vi "诊断标定3 - 副本.vi"(8 "CAN端口":u16(ring), 9 "设备索引号":u16(ring), 10 "CAN卡类型":u32(ring)=21) -> ()   [LabVIEW 2013] (continued)
        }
        n2820 = Unbundle By Name(w898) -> ("status"=w897:bool)
        n2821 = Or(x=w897, y=w899) -> (x .or. y?=w900:bool)
      }
      n2822 = Release Queue(queue=w893, force destroy? (F)=TRUE ("强制销毁？(F)"), error in (no error)=w892) -> (error out=w890:errorcluster)  [unwired: 2 out]
      n2823 = call <vilib>:"Clear Errors.vi"("error in (no error)"=w890) -> ()  [unwired: 7 out]
    }
    frame Disabled {
    }
  }
  n2824 = while {
    tunnel: w36 -> [w3698]
    tunnel: w35 -> [w3697]
    tunnel: [w3696] -> w39
    tunnel: [w3695] -> w38
    tunnel: w31 -> [_]
    tunnel: w34 -> [w3687]
    stop <- w3694 stop-if-true
    n2825 = local read "停止"() -> (w3694:bool)
    n2826 = local read "设备索引号"() -> (w3691:u16)
    n2827 = local read "CAN卡类型"() -> (w3692:u32)
    n2828 = local read "CAN端口"() -> (w3690:u16)
    n2829 = call "receiver-8.6.vi"("错误输入（无错误）"=w3687, "CAN端口"=w3690, "设备索引号"=w3691, "CAN卡类型"=w3692) -> ("错误输出"=w3693:errorcluster, "输出簇"=w3689:T25, "接收成功"=w3688:bool)  [unwired: 3 out]
    n2830 = call <vilib>:"Clear Errors.vi"("error in (no error)"=w3693) -> ()  [unwired: 6 in, 1 out]
    n2831 = case shown="真" w3688 {
      tunnel: w3697 -> [w3699 w3705]
      tunnel: w3689 -> [_ w3704]
      tunnel: w3698 -> [w3700 w3703]
      tunnel: [w3700 w3702] -> w3696
      tunnel: [w3699 w3701] -> w3695
      frame False {
      }
      frame True {
        n2832 = Enqueue Element(queue=w3703, element=w3704, error in (no error)=w3705) -> (queue out=w3702:refnum<queue>, error out=w3701:errorcluster)  [unwired: 2 out]
      }
    }
  }
  n2833 = while {
    tunnel: w36 -> [w3713]
    tunnel: w35 -> [w3712]
    stop <- w3706 stop-if-true
    n2834 = local read "停止"() -> (w3706:bool)
    n2835 = local read "控制1"() -> (w3708:bool)
    n2836 = Dequeue Element(queue=w3713, timeout in ms (-1)=200 ("超时毫秒(-1)"), error in (no error)=w3712) -> (element=w3711:T3, error out=w3710:errorcluster)  [unwired: 2 out]
    n2837 = case shown="无错误" w3710 {
      tunnel: w3711 -> [w3718 _]
      tunnel: "写?" -> [w3715 _]
      tunnel: w3708 -> [w3714 _]
      frame No Error {
        n2838 = Unbundle(w3718) -> ("return type"=w3717:u32, "pReceive"=w3716:T26)
        n2839 = for {
          N: w3717 -> [_]
          tunnel: w3716 -> [w3722] mode=indexing
          tunnel: w3715 -> [w3720]
          tunnel: w3714 -> [w3719]
          n2840 = Unbundle By Name(w3722) -> ("ID"=w3723:u32)
          n2841 = call "ID解析.vi"("ID"=w3723) -> ("PDU(1)"=w3721:i32)  [unwired: 10 out]
          n2842 = case shown="18" w3721 {
            tunnel: w3722 -> [_ w3733]
            tunnel: w3720 -> [_ w3725]
            tunnel: w3719 -> [_ w3724]
            frame 0, Default {
            }
            frame 24 {
              n2843 = local read "主从选择"() -> (w3726:enum32{"主板", "从板"})
              n2844 = local read "设备索引号"() -> (w3729:u16)
              n2845 = local read "CAN卡类型"() -> (w3728:u32)
              n2846 = local read "CAN端口"() -> (w3730:u16)
              n2847 = disable-structure shown="禁用" {
                disable-tunnel: w3733 -> [w3736 _]
                frame Disabled {
                  n2848 = call "标定授权读取.vi"("VCI_Receive"=w3736) -> ()  [unwired: 1 out]
                }
                frame Enabled {
                }
              }
              n2849 = case shown="\"从板\"" w3726 {
                tunnel: [0 ("FUNC") w3735] -> w3727
                frame "主板", Default {
                }
                frame "从板" {
                  n2850 = local read "从板号"() -> (w3735:u8)
                }
              }
              n2851 = local read "面板选择"() -> (w3732:T7)
              n2852 = case shown="\"读写参数\", 默认" w3732 {
                tunnel: w3725 -> [w3741 _ _ _]
                tunnel: "命令" -> [w3742 w3841 w4096 w4236]
                tunnel: w3726 -> [w3751 _ w4104 w4244]
                tunnel: w3733 -> [_ _ _ _]
                tunnel: w3733 -> [w3747 w3842 w4098 w4238]
                tunnel: w3730 -> [w3746 w3843 w4099 w4239]
                tunnel: w3729 -> [w3745 w3844 w4100 w4240]
                tunnel: w3728 -> [w3744 w3845 w4101 w4241]
                tunnel: w3727 -> [w3743 _ w4097 w4237]
                tunnel: w3724 -> [w3737 _ _ _]
                frame "读写参数", Default {
                  n2853 = local read "命令序号"() -> (w3740:u8)
                  n2854 = call "多帧接收机制(EV05).vi"("can卡类型"=w3744, "设备索引号"=w3745, "CAN端口"=w3746, "VCI_Receive"=w3747, "命令"=w3742, "板号"=w3743, "写?"=w3741, "命令序号"=w3740) -> ("错误信号"=w3738:bool, "错误代码"=w3750:i32, "输出数组"=w3749:u8[], "读错误代码"=w3739:u8[], "结束信号"=w3748:bool)  [unwired: 7 out]
                  n2855 = case shown="假" w3741 {
                    tunnel: w3748 -> [w3761 w3824]
                    tunnel: w3750 -> [w3760 w3823]
                    tunnel: w3740 -> [w3759 _]
                    tunnel: w3749 -> [w3758 _]
                    tunnel: w3742 -> [w3757 _]
                    tunnel: w3751 -> [w3755 w3822]
                    tunnel: w3739 -> [w3754 _]
                    tunnel: w3738 -> [w3753 _]
                    tunnel: w3737 -> [w3752 _]
                    frame False {
                      # "读参数"
                      n2856 = And(x=w3752, y=w3761) -> (x .and. y?=w3756:bool)
                      n2857 = case shown="真" w3756 {
                        tunnel: w3760 -> [_ w3772]
                        tunnel: w3759 -> [_ w3771]
                        tunnel: w3758 -> [_ w3770]
                        tunnel: w3757 -> [_ w3769]
                        tunnel: w3755 -> [_ w3765]
                        tunnel: w3754 -> [_ w3763]
                        tunnel: w3753 -> [_ w3764]
                        frame False {
                        }
                        frame True {
                          n2858 = case shown="假" w3764 {
                            tunnel: w3772 -> [w3781 _]
                            tunnel: w3771 -> [w3780 _]
                            tunnel: w3770 -> [w3779 _]
                            tunnel: w3769 -> [w3777 _]
                            tunnel: w3765 -> [w3773 _]
                            tunnel: w3763 -> [_ w3807]
                            frame False {
                              n2859 = case shown="\"主板\", 默认" w3773 {
                                tunnel: [w3782 _] -> w3776
                                tunnel: [_ w3795] -> w3775
                                frame "主板", Default {
                                n2860 = stacked-sequence {
                                tunnel: [_ w3794] -> w3782
                                frame #0 {
                                n2861 = control-ref of="一级故障"() -> (w3788:refnum<vi>)
                                n2862 = control-ref of="一级故障 2"() -> (w3790:refnum<vi>)
                                n2863 = control-ref of="一级故障 3"() -> (w3791:refnum<vi>)
                                n2864 = control-ref of="加热控制参数"() -> (w3792:refnum<vi>)
                                n2865 = control-ref of="充电控制参数"() -> (w3793:refnum<vi>)
                                n2866 = control-ref of="电池信息"() -> (w3786:refnum<vi>)
                                n2867 = control-ref of="项目信息"() -> (w3789:refnum<vi>)
                                n2868 = control-ref of="项目信息2"() -> (w3787:refnum<vi>)
                                n2869 = control-ref of="高压参数"() -> (w3785:refnum<vi>)
                                n2870 = local read "主板数据"() -> (w3784:T4)
                                n2871 = Bundle(cluster=w3784, "项目信息"=w3789, "一级故障 4"=w3787, "一级故障"=w3788, "一级故障 2"=w3790, "一级故障 3"=w3791, "加热控制参数"=w3792, "充电控制参数"=w3793, "高压参数"=w3785, "电池信息"=w3786) -> (w3783:T4)
                                n2872 = local write "主板数据"(w3783) -> ()
                                }
                                frame #1 {
                                n2873 = control-ref of="主板数据"() -> (w3794:refnum<vi>)
                                }
                                }
                                }
                                frame "从板" {
                                n2874 = stacked-sequence {
                                tunnel: [_ w3806] -> w3795
                                frame #0 {
                                n2875 = control-ref of="从板号"() -> (w3800:refnum<vi>)
                                n2876 = control-ref of="项目信息 2"() -> (w3801:refnum<vi>)
                                n2877 = control-ref of="电池组信息"() -> (w3799:refnum<vi>)
                                n2878 = control-ref of="加热控制参数"() -> (w3802:refnum<vi>)
                                n2879 = control-ref of="一级故障(从板)"() -> (w3803:refnum<vi>)
                                n2880 = control-ref of="二级故障(从板)"() -> (w3804:refnum<vi>)
                                n2881 = control-ref of="三级故障(从板)"() -> (w3805:refnum<vi>)
                                n2882 = control-ref of="均衡参数"() -> (w3798:refnum<vi>)
                                n2883 = local read "从板信息"() -> (w3797:T2)
                                n2884 = Bundle(cluster=w3797, "从板号"=w3800, "项目信息 2"=w3801, "加热控制参数"=w3802, "一级故障(从板)"=w3803, "二级故障(从板)"=w3804, "三级故障(从板)"=w3805, "电池组信息(从板)"=w3799, "均衡参数"=w3798) -> (w3796:T2)
                                n2885 = local write "从板信息"(w3796) -> ()
                                }
                                frame #1 {
                                n2886 = control-ref of="从板信息"() -> (w3806:refnum<vi>)
                                }
                                }
                                }
                              }
                              n2887 = control-ref of="结果"() -> (w3778:refnum<vi>)
                              n2888 = control-ref of="从板个数"() -> (w3774:refnum<vi>)
                              n2889 = call "输出数据解析.vi"("主板引用"=w3776, "从板引用"=w3775, "板选择"=w3773, "错误代码"=w3781, "命令序号"=w3780, "输入数组"=w3779, "命令"=w3777, "进度引用"=w3778, "从板个数"=w3774) -> ()  [unwired: 2 in, 5 out]
                            }
                            frame True {
                              n2890 = Index Array(array=w3807, index #1=0 ("索引"), index #2=1 ("索引")) -> (element #1=w3810:u8, element #2=w3811:u8)
                              n2891 = Join Numbers(hi=w3810, lo=w3811) -> ((hi.lo)=w3809:u16)
                              n2892 = Number To Hexadecimal String(2:w3809) -> (0:w3808:string)  [unwired: 1 out]
                              n2893 = control-ref of="结果"() -> (w3816:refnum<vi>)
                              n2894 = Concatenate Strings("0x" ("字符串"), w3808) -> (w3817:string)
                              n2895 = Build Array(w3817) -> (w3818:string[])
                              n2896 = call "表格编辑.vi"("新元素/子数组"=w3818, "活动单元格:单元格背景色"=u32 16740749, "MCListbox引用句柄"=w3816) -> ()  [unwired: 9 out]
                            }
                          }
                          n2897 = global write "EV05全局变量1.vi" "流控帧 2"(FALSE ("流控帧 2")) -> ()
                          n2898 = global write "EV05全局变量1.vi" "输出数组"(i32[] []) -> ()
                          n2899 = local write "控制1"(FALSE ("控制1")) -> ()
                          n2900 = local write "消除"(FALSE ("消除")) -> ()
                        }
                      }
                    }
                    frame True {
                      # "写参数判定"
                      n2901 = And(x="控制1", y=w3824) -> (x .and. y?=w3821:bool)
                      n2902 = case shown="真" w3821 {
                        tunnel: w3823 -> [_ w3831]
                        tunnel: w3822 -> [_ w3828]
                        frame False {
                        }
                        frame True {
                          n2903 = call <vilib>:"Unset Busy.vi"() -> ()  [unwired: 2 in, 10 out]
                          n2904 = case shown="\"从板\"" w3828 {
                            tunnel: [w3832 w3833] -> w3830
                            frame "主板", Default {
                              n2905 = local read "主板选项"() -> (w3832:string)
                            }
                            frame "从板" {
                              n2906 = local read "从板选项"() -> (w3833:string)
                            }
                          }
                          n2907 = control-ref of="结果"() -> (w3829:refnum<vi>)
                          n2908 = call "输入数据判定.vi"("主从选择"=w3828, "主板选项"=w3830, "进度引用"=w3829, "错误代码"=w3831) -> ()  [unwired: 2 in, 6 out]
                          n2909 = global write "EV05全局变量1.vi" "流控帧 2"(FALSE ("流控帧 2")) -> ()
                          n2910 = local write "控制1"(FALSE ("控制1")) -> ()
                          n2911 = local write "消除"(FALSE ("消除")) -> ()
                        }
                      }
                      n2912 = global write "EV05全局变量1.vi" "输出数组"(i32[] []) -> ()
                    }
                  }
                }
                frame "版本读取" {
                  n2913 = local read "命令序号"() -> (w3834:u8)
                  n2914 = local read "从板板号"() -> (w3837:u8)
                  n2915 = local read "控制1"() -> (w3838:bool)
                  n2916 = call "多帧接收机制(EV05).vi"("can卡类型"=w3845, "设备索引号"=w3844, "CAN端口"=w3843, "VCI_Receive"=w3842, "命令"=w3841, "板号"=w3837, "命令序号"=w3834) -> ("错误信号"=w3835:bool, "输出数组"=w3846:u8[], "读错误代码"=w3836:u8[], "结束信号"=w3840:bool)  [unwired: 1 in, 8 out]
                  n2917 = And(x=w3838, y=w3840) -> (x .and. y?=w3839:bool)
                  n2918 = case shown="真" w3839 {
                    tunnel: w3846 -> [_ w3854]
                    tunnel: w3834 -> [_ w3853]
                    tunnel: w3841 -> [_ w3852]
                    tunnel: w3836 -> [_ w3848]
                    tunnel: w3835 -> [_ w3847]
                    frame False {
                    }
                    frame True {
                      n2919 = case shown="假" w3847 {
                        tunnel: w3854 -> [w3858 _]
                        tunnel: w3853 -> [w3857 _]
                        tunnel: w3852 -> [w3856 _]
                        tunnel: w3848 -> [w3855 w4082]
                        frame False {
                          n2920 = case shown="89" w3856 {
                            tunnel: w3857 -> [_ w3861]
                            tunnel: w3858 -> [_ w3860]
                            tunnel: w3855 -> [_ _]
                            frame 0, Default {
                            }
                            frame 137 {
                              n2921 = case shown="1" w3861 {
                                tunnel: w3860 -> [_ w3889 w3933 w3953 w4080]
                                frame 0, Default {
                                }
                                frame 1 {
                                w3871 = "." ("字符串")
                                n2922 = Array Subset(array=w3889, index=0 ("索引"), length=14 ("长度")) -> (w3902:u8[])
                                n2923 = Index Array(array=w3889, index=14 ("索引")) -> (element=w3892:u8)
                                n2924 = Index Array(array=w3889, index #1=15 ("索引"), index #2=16 ("索引")) -> (element #1=w3898:u8, element #2=w3899:u8)
                                n2925 = Index Array(array=w3889, index #1=17 ("索引"), index #2=18 ("索引")) -> (element #1=w3893:u8, element #2=w3894:u8)
                                n2926 = call "数组去零.vi"("输入"=w3902) -> ("输出"=w3877:dbl[])
                                n2927 = Join Numbers(hi=w3893, lo=w3894) -> ((hi.lo)=w3890:u16)
                                n2928 = Join Numbers(hi=w3898, lo=w3899) -> ((hi.lo)=w3891:u16)
                                n2929 = Number To Decimal String(number=w3892) -> (decimal integer string=w3884:string)  [unwired: 1 out]
                                n2930 = Byte Array To String(unsigned byte array=w3877) -> (string=w3876:string)
                                n2931 = Number To Decimal String(number=w3890) -> (decimal integer string=w3872:string)  [unwired: 1 out]
                                n2932 = Number To Decimal String(number=w3891) -> (decimal integer string=w3883:string)  [unwired: 1 out]
                                n2933 = Array Subset(array=w3889, index=21 ("索引"), length=7 ("长度")) -> (w3886:u8[])
                                n2934 = Concatenate Strings("V" ("字符串"), w3884, w3871, w3883, w3871, w3872) -> (w3881:string)
                                n2935 = call "数组去零.vi"("输入"=w3886) -> ("输出"=w3869:dbl[])
                                n2936 = Byte Array To String(unsigned byte array=w3869) -> (string=w3867:string)
                                n2937 = call <vilib>:"Space Constant.vi"() -> ("String"=w3868:string)
                                n2938 = Equal?(x=w3867, y=w3868) -> (x = y?=w3873:bool)
                                n2939 = Concatenate Strings("-" ("字符串"), w3867) -> (w3874:string)
                                n2940 = Select(t=w3868, s=w3873, f=w3874) -> (s? t:f=w3870:string)
                                n2941 = Concatenate Strings(w3876, "-" ("字符串"), w3881, w3870) -> (w3863:string)
                                n2942 = local read "项目软件版本"() -> (w3865:string[])
                                n2943 = local read "从板板号"() -> (w3862:u8)
                                n2944 = local write "项目软件版本号"(w3863) -> ()
                                n2945 = Replace Array Subset(array=w3865, new element=w3863, index=w3862) -> (w3864:string[])
                                n2946 = control-ref of="结果"() -> (w3880:refnum<vi>)
                                n2947 = local write "项目软件版本"(w3864) -> ()
                                n2948 = Build Array("项目软件版本     读取完成" ("读取结果")) -> (w3878:string[])
                                n2949 = call "表格编辑(版本读取).vi"("新元素/子数组"=w3878, "活动单元格:单元格背景色"=u32 6618880, "MCListbox引用句柄"=w3880) -> ()  [unwired: 9 out]
                                }
                                frame 2 {
                                w3916 = ""
                                w3913 = "." ("字符串")
                                n2950 = Array Subset(array=w3933, index=0 ("索引"), length=14 ("长度")) -> (w3921:u8[])
                                n2951 = Index Array(array=w3933, index=14 ("索引")) -> (element=w3936:u8)
                                n2952 = Index Array(array=w3933, index #1=15 ("索引"), index #2=16 ("索引")) -> (element #1=w3942:u8, element #2=w3943:u8)
                                n2953 = Index Array(array=w3933, index #1=17 ("索引"), index #2=18 ("索引")) -> (element #1=w3937:u8, element #2=w3938:u8)
                                n2954 = Join Numbers(hi=w3937, lo=w3938) -> ((hi.lo)=w3934:u16)
                                n2955 = Join Numbers(hi=w3942, lo=w3943) -> ((hi.lo)=w3935:u16)
                                n2956 = Number To Decimal String(number=w3934) -> (decimal integer string=w3914:string)  [unwired: 1 out]
                                n2957 = call "数组去零.vi"("输入"=w3921) -> ("输出"=w3920:dbl[])
                                n2958 = Number To Decimal String(number=w3936) -> (decimal integer string=w3928:string)  [unwired: 1 out]
                                n2959 = Number To Decimal String(number=w3935) -> (decimal integer string=w3927:string)  [unwired: 1 out]
                                n2960 = Array Subset(array=w3933, index=21 ("索引"), length=7 ("长度")) -> (w3930:u8[])
                                n2961 = Byte Array To String(unsigned byte array=w3920) -> (string=w3915:string)
                                n2962 = call "数组去零.vi"("输入"=w3930) -> ("输出"=w3912:dbl[])
                                n2963 = Concatenate Strings("V" ("字符串"), w3928, w3913, w3927, w3913, w3914) -> (w3925:string)
                                n2964 = Byte Array To String(unsigned byte array=w3912) -> (string=w3910:string)
                                n2965 = Equal?(x=w3916, y=w3910) -> (x = y?=w3917:bool)
                                n2966 = Concatenate Strings("-" ("字符串"), w3910) -> (w3918:string)
                                n2967 = Select(t=w3916, s=w3917, f=w3918) -> (s? t:f=w3911:string)
                                n2968 = Concatenate Strings(w3915, "-" ("字符串"), w3925, w3911) -> (w3906:string)
                                n2969 = local read "平台软件版本"() -> (w3908:string[])
                                n2970 = local read "从板板号"() -> (w3905:u8)
                                n2971 = local write "平台软件版本号"(w3906) -> ()
                                n2972 = Replace Array Subset(array=w3908, new element=w3906, index=w3905) -> (w3907:string[])
                                n2973 = control-ref of="结果"() -> (w3923:refnum<vi>)
                                n2974 = local write "平台软件版本"(w3907) -> ()
                                n2975 = Build Array("平台软件版本     读取完成" ("读取结果")) -> (w3922:string[])
                                n2976 = call "表格编辑(版本读取).vi"("新元素/子数组"=w3922, "活动单元格:单元格背景色"=u32 6618880, "MCListbox引用句柄"=w3923) -> ()  [unwired: 1 in, 8 out]
                                }
                                frame 3 {
                                n2977 = Index Array(array=w3953, index #1=0 ("索引"), index #2=1 ("索引")) -> (element #1=w3949:u8, element #2=w3950:u8)
                                n2978 = Join Numbers(hi=w3949, lo=w3950) -> ((hi.lo)=w3948:u16)
                                n2979 = case shown="99, 默认" w3948 {
                                tunnel: w3953 -> [w3956 _ w3990]
                                tunnel: w3948 -> [_ _ w3968]
                                frame 0 {
                                n2980 = Index Array(array=w3956, index #1=2 ("索引"), index #2=3 ("索引")) -> (element #1=w3960:u8, element #2=w3959:u8)
                                n2981 = Join Numbers(hi=w3960, lo=w3959) -> ((hi.lo)=w3955:u16)
                                n2982 = for {
                                N: w3955 -> [_]
                                tunnel: w3956 -> [w3965]
                                tunnel: [w3961] -> w3954 mode=indexing
                                i -> [w3964]
                                n2983 = Add(x=w3964, y=4) -> (x+y=w3962:i32)
                                n2984 = Index Array(array=w3965, index=w3962) -> (element=w3961:u8)
                                }
                                "MODEL号" <- w3954
                                }
                                frame 99, Default {
                                }
                                frame 1..40 {
                                w3973 = ""
                                w3994 = "." ("字符串")
                                n2985 = Array Subset(array=w3990, index=2 ("索引"), length=14 ("长度")) -> (w3979:u8[])
                                n2986 = Index Array(array=w3990, index=16 ("索引")) -> (element=w4002:u8)
                                n2987 = Index Array(array=w3990, index #1=17 ("索引"), index #2=18 ("索引")) -> (element #1=w4008:u8, element #2=w4009:u8)
                                n2988 = Index Array(array=w3990, index #1=19 ("索引"), index #2=20 ("索引")) -> (element #1=w4003:u8, element #2=w4004:u8)
                                n2989 = Join Numbers(hi=w4003, lo=w4004) -> ((hi.lo)=w4000:u16)
                                n2990 = Join Numbers(hi=w4008, lo=w4009) -> ((hi.lo)=w4001:u16)
                                n2991 = Number To Decimal String(number=w3968) -> (decimal integer string=w3988:string)  [unwired: 1 out]
                                n2992 = Number To Decimal String(number=w4002) -> (decimal integer string=w3996:string)  [unwired: 1 out]
                                n2993 = call "数组去零.vi"("输入"=w3979) -> ("输出"=w3978:dbl[])
                                n2994 = Number To Decimal String(number=w4001) -> (decimal integer string=w3995:string)  [unwired: 1 out]
                                n2995 = Number To Decimal String(number=w4000) -> (decimal integer string=w3993:string)  [unwired: 1 out]
                                n2996 = Byte Array To String(unsigned byte array=w3978) -> (string=w3980:string)
                                n2997 = Concatenate Strings("第" ("读取结果"), w3988, "模块" ("字符串"), "     读取完成" ("读取结果")) -> (w3981:string)
                                n2998 = Concatenate Strings("V" ("字符串"), w3996, w3994, w3995, w3994, w3993) -> (w3991:string)
                                n2999 = control-ref of="结果"() -> (w3984:refnum<vi>)
                                n3000 = Array Subset(array=w3990, index=23 ("索引"), length=7 ("长度")) -> (w3977:u8[])
                                n3001 = call "数组去零.vi"("输入"=w3977) -> ("输出"=w3972:dbl[])
                                n3002 = Byte Array To String(unsigned byte array=w3972) -> (string=w3969:string)
                                n3003 = Build Array(w3981) -> (w3983:string[])
                                n3004 = control-ref of="模块软件版本 2"() -> (w3985:refnum<vi>)
                                n3005 = local read "模块软件版本"() -> (w3986:T1)
                                n3006 = Equal?(x=w3973, y=w3969) -> (x = y?=w3974:bool)
                                n3007 = call "表格编辑(版本读取).vi"("新元素/子数组"=w3983, "活动单元格:单元格背景色"=u32 6618880, "MCListbox引用句柄"=w3984) -> ()  [unwired: 1 in, 8 out]
                                n3008 = Concatenate Strings("-" ("字符串"), w3969) -> (w3975:string)
                                n3009 = Select(t=w3973, s=w3974, f=w3975) -> (s? t:f=w3971:string)
                                n3010 = Concatenate Strings(w3980, "-" ("字符串"), w3991, w3971) -> (w3970:string)
                                n3011 = case shown="30" w3968 {
                                tunnel: [_ "VERSIONM" "BCUMCAL" "BMUMCAL" "BMURMCAL" "BCUCMCAL" "BCUDMCAL" "SCH" "BSW" "CDD" "DATALAYER" "DATAANALYSIS" "SOC" "SOH" "SOF" "INTRES" "INTCAN" "CARCAN" "CHGCANL" "THM" "CHGM" "HVM" "LVM" "BALM" "SAFEM" "RUNMODEM" "RELAY" "DO" "GBCHGDET" "SUPPLYPOWGDET" "SUMVDET" "CURDET" "TEMPERDET" "CELLVDET" "ISODET" "AI" "DI" "SYSCONF" "ECUCONF"] -> w3967
                                frame 0, Default {
                                }
                                frame 1 {
                                }
                                frame 2 {
                                }
                                frame 3 {
                                }
                                frame 4 {
                                }
                                frame 5 {
                                }
                                frame 6 {
                                }
                                frame 7 {
                                }
                                frame 8 {
                                }
                                frame 9 {
                                }
                                frame 10 {
                                }
                                frame 11 {
                                }
                                frame 12 {
                                }
                                frame 13 {
                                }
                                frame 14 {
                                }
                                frame 15 {
                                }
                                frame 16 {
                                }
                                frame 17 {
                                }
                                frame 18 {
                                }
                                frame 19 {
                                }
                                frame 20 {
                                }
                                frame 21 {
                                }
                                frame 22 {
                                }
                                frame 23 {
                                }
                                frame 24 {
                                }
                                frame 25 {
                                }
                                frame 26 {
                                }
                                frame 27 {
                                }
                                frame 28 {
                                }
                                frame 29 {
                                }
                                frame 30 {
                                }
                                frame 31 {
                                }
                                frame 32 {
                                }
                                frame 33 {
                                }
                                frame 34 {
                                }
                                frame 35 {
                                }
                                frame 36 {
                                }
                                frame 37 {
                                }
                                frame 38 {
                                }
                                }
                                n3012 = case shown="\"全部读取\"" w3986 {
                                tunnel: w3970 -> [w4053 w4061]
                                tunnel: w3968 -> [w4057 w4066]
                                tunnel: w3985 -> [w4059 w4067]
                                tunnel: w3967 -> [w4058 w4065]
                                frame "全部读取" {
                                n3013 = Number To Decimal String(number=w4057) -> (decimal integer string=w4056:string)  [unwired: 1 out]
                                n3014 = Concatenate Strings(w4056, "-" ("元素"), w4058) -> (w4054:string)
                                n3015 = Build Array(w4054, w4053) -> (w4052:string[])
                                n3016 = call "表格编辑(模块版本).vi"("新元素/子数组"=w4052, "MCListbox引用句柄"=w4059) -> ()  [unwired: 1 in, 9 out]
                                }
                                frame "BCUMCAL", Default {
                                n3017 = Number To Decimal String(number=w4066) -> (decimal integer string=w4064:string)  [unwired: 1 out]
                                n3018 = Concatenate Strings(w4064, "-" ("元素"), w4065) -> (w4062:string)
                                n3019 = Build Array(w4062, w4061) -> (w4060:string[])
                                n3020 = call "表格编辑(模块版本).vi"("新元素/子数组"=w4060, "MCListbox引用句柄"=w4067) -> ()  [unwired: 1 in, 9 out]
                                }
                                }
                                }
                                }
                                }
                                frame 4 {
                                n3021 = Array Subset(array=w4080, length=12 ("长度")) -> (w4078:u8[])  [unwired: 1 in]
                                n3022 = Byte Array To String(unsigned byte array=w4078) -> (string=w4077:string)
                                n3023 = call <vilib>:"Trim Whitespace.vi"("string"=w4077) -> ("trimmed string"=w4069:string)  [unwired: 1 in]
                                n3024 = local read "从板板号"() -> (w4068:u8)
                                n3025 = local write "硬件版本号"(w4069) -> ()
                                n3026 = local read "硬件版本"() -> (w4070:string[])
                                n3027 = Replace Array Subset(array=w4070, new element=w4069, index=w4068) -> (w4071:string[])
                                n3028 = local write "硬件版本"(w4071) -> ()
                                n3029 = global write "EV05全局变量1.vi" "写入超时"(TRUE ("写入超时")) -> ()
                                n3030 = control-ref of="结果"() -> (w4075:refnum<vi>)
                                n3031 = Build Array("硬件版本     读取完成" ("读取结果")) -> (w4074:string[])
                                n3032 = call "表格编辑(版本读取).vi"("新元素/子数组"=w4074, "活动单元格:单元格背景色"=u32 6618880, "MCListbox引用句柄"=w4075) -> ()  [unwired: 9 out]
                                }
                              }
                              n3033 = global write "EV05全局变量1.vi" "写入超时"(TRUE ("写入超时")) -> ()
                            }
                          }
                        }
                        frame True {
                          n3034 = Index Array(array=w4082, index #1=0 ("索引"), index #2=1 ("索引")) -> (element #1=w4087:u8, element #2=w4088:u8)
                          n3035 = Join Numbers(hi=w4087, lo=w4088) -> ((hi.lo)=w4086:u16)
                          n3036 = Number To Hexadecimal String(2:w4086) -> (0:w4085:string)  [unwired: 1 out]
                          n3037 = control-ref of="结果"() -> (w4084:refnum<vi>)
                          n3038 = Concatenate Strings("0x" ("字符串"), w4085) -> (w4092:string)
                          n3039 = Build Array(w4092) -> (w4083:string[])
                          n3040 = call "表格编辑(版本读取).vi"("新元素/子数组"=w4083, "活动单元格:单元格背景色"=u32 16740749, "MCListbox引用句柄"=w4084) -> ()  [unwired: 9 out]
                        }
                      }
                      n3041 = global write "EV05全局变量1.vi" "流控帧 2"(FALSE ("流控帧 2")) -> ()
                      n3042 = local write "控制1"(FALSE ("控制1")) -> ()
                      n3043 = local write "消除"(FALSE ("消除")) -> ()
                      n3044 = call <vilib>:"Unset Busy.vi"() -> ()  [unwired: 2 in, 10 out]
                    }
                  }
                }
                frame "其它诊断" {
                  n3045 = local read "命令序号"() -> (w4094:u8)
                  n3046 = call "多帧接收机制(EV05).vi"("can卡类型"=w4101, "设备索引号"=w4100, "CAN端口"=w4099, "VCI_Receive"=w4098, "命令"=w4096, "板号"=w4097, "命令序号"=w4094) -> ("错误代码"=w4103:i32, "输出数组"=w4095:u8[], "读错误代码"=w4093:u8[], "结束信号"=w4102:bool)  [unwired: 1 in, 8 out]
                  n3047 = case shown="真" w4102 {
                    tunnel: w4104 -> [_ w4105]
                    tunnel: w4103 -> [_ _]
                    tunnel: w4095 -> [_ w4106]
                    tunnel: w4094 -> [_ w4109]
                    tunnel: w4093 -> [_ w4107]
                    frame False {
                    }
                    frame True {
                      n3048 = Insert Into Array(array=w4107, new element=w4106) -> (w4108:u8[])  [unwired: 1 in]
                      n3049 = case shown="1" w4109 {
                        tunnel: w4108 -> [_ w4118 w4204]
                        tunnel: w4105 -> [_ _ w4199]
                        frame 0, Default {
                        }
                        frame 1 {
                          n3050 = Index Array(array=w4118) -> (element #1=w4117:u8, element #2=w4116:u8, element #3=w4115:u8)  [unwired: 3 in]
                          n3051 = Join Numbers(hi=w4116, lo=w4115) -> ((hi.lo)=w4114:u16)
                          n3052 = case shown="4" w4117 {
                            tunnel: w4118 -> [_ _ _ _ _ _ _ _ _ _]
                            tunnel: w4114 -> [_ w4121 w4129 w4139 w4149 w4159 w4169 w4179 w4189 _]
                            frame 0, Default {
                              n3053 = local write "继电器超时处理"(FALSE ("继电器超时处理")) -> ()
                            }
                            frame 1 {
                              n3054 = Equal To 0?(x=w4121) -> (x = 0?=w4120:bool)
                              n3055 = local write "正级继电器 12"(w4120) -> ()
                              n3056 = case shown="假" w4120 {
                                tunnel: w4121 -> [w4124 _]
                                frame False {
                                n3057 = local read "正级继电器"() -> (w4126:bool)
                                n3058 = Number To Hexadecimal String(2:w4124) -> (0:w4123:string)  [unwired: 1 out]
                                n3059 = local write "继电器超时处理"(TRUE ("继电器超时处理")) -> ()
                                n3060 = Not(x=w4126) -> (.not. x?=w4125:bool)
                                n3061 = Concatenate Strings("继电器操作失败,0x" ("消息"), w4123) -> ()  [unwired: 1 out]
                                n3062 = local write "正级继电器"(w4125) -> ()
                                }
                                frame True {
                                (unwired) "继电器操作成功!\n继电器操作成功!\n继电器操作成功!"
                                }
                              }
                            }
                            frame 2 {
                              n3063 = Equal To 0?(x=w4129) -> (x = 0?=w4128:bool)
                              n3064 = case shown="假" w4128 {
                                tunnel: w4129 -> [w4135 _]
                                tunnel: [w4133 "继电器操作成功!\n继电器操作成功!\n继电器操作成功!"] -> _
                                frame False {
                                n3065 = local read "负级继电器"() -> (w4131:bool)
                                n3066 = Number To Hexadecimal String(2:w4135) -> (0:w4134:string)  [unwired: 1 out]
                                n3067 = local write "继电器超时处理"(TRUE ("继电器超时处理")) -> ()
                                n3068 = Not(x=w4131) -> (.not. x?=w4132:bool)
                                n3069 = Concatenate Strings("继电器操作失败,0x" ("消息"), w4134) -> (w4133:string)
                                n3070 = local write "负级继电器"(w4132) -> ()
                                }
                                frame True {
                                }
                              }
                              n3071 = local write "正级继电器 2"(w4128) -> ()
                            }
                            frame 3 {
                              n3072 = Equal To 0?(x=w4139) -> (x = 0?=w4138:bool)
                              n3073 = case shown="假" w4138 {
                                tunnel: w4139 -> [w4145 _]
                                tunnel: [w4143 "继电器操作成功!\n继电器操作成功!\n继电器操作成功!"] -> _
                                frame False {
                                n3074 = local read "预充电继电器"() -> (w4141:bool)
                                n3075 = Number To Hexadecimal String(2:w4145) -> (0:w4144:string)  [unwired: 1 out]
                                n3076 = local write "继电器超时处理"(TRUE ("继电器超时处理")) -> ()
                                n3077 = Not(x=w4141) -> (.not. x?=w4142:bool)
                                n3078 = Concatenate Strings("继电器操作失败,0x" ("消息"), w4144) -> (w4143:string)
                                n3079 = local write "预充电继电器"(w4142) -> ()
                                }
                                frame True {
                                }
                              }
                              n3080 = local write "正级继电器 3"(w4138) -> ()
                            }
                            frame 4 {
                              n3081 = Equal To 0?(x=w4149) -> (x = 0?=w4148:bool)
                              n3082 = case shown="假" w4148 {
                                tunnel: w4149 -> [w4155 _]
                                tunnel: [w4153 "继电器操作成功!\n继电器操作成功!\n继电器操作成功!"] -> _
                                frame False {
                                n3083 = local read "加热继电器"() -> (w4152:bool)
                                n3084 = Number To Hexadecimal String(2:w4155) -> (0:w4154:string)  [unwired: 1 out]
                                n3085 = local write "继电器超时处理"(TRUE ("继电器超时处理")) -> ()
                                n3086 = Not(x=w4152) -> (.not. x?=w4151:bool)
                                n3087 = Concatenate Strings("继电器操作失败,0x" ("消息"), w4154) -> (w4153:string)
                                n3088 = local write "加热继电器"(w4151) -> ()
                                }
                                frame True {
                                }
                              }
                              n3089 = local write "正级继电器 5"(w4148) -> ()
                            }
                            frame 5 {
                              n3090 = Equal To 0?(x=w4159) -> (x = 0?=w4158:bool)
                              n3091 = case shown="假" w4158 {
                                tunnel: w4159 -> [w4165 _]
                                tunnel: [w4163 "继电器操作成功!\n继电器操作成功!\n继电器操作成功!"] -> _
                                frame False {
                                n3092 = local read "充电继电器"() -> (w4161:bool)
                                n3093 = Number To Hexadecimal String(2:w4165) -> (0:w4164:string)  [unwired: 1 out]
                                n3094 = local write "继电器超时处理"(TRUE ("继电器超时处理")) -> ()
                                n3095 = Not(x=w4161) -> (.not. x?=w4162:bool)
                                n3096 = Concatenate Strings("继电器操作失败,0x" ("消息"), w4164) -> (w4163:string)
                                n3097 = local write "充电继电器"(w4162) -> ()
                                }
                                frame True {
                                }
                              }
                              n3098 = local write "正级继电器 4"(w4158) -> ()
                            }
                            frame 6 {
                              n3099 = Equal To 0?(x=w4169) -> (x = 0?=w4168:bool)
                              n3100 = local write "正级继电器 6"(w4168) -> ()
                              n3101 = case shown="假" w4168 {
                                tunnel: w4169 -> [w4175 _]
                                tunnel: [w4173 "继电器操作成功!\n继电器操作成功!\n继电器操作成功!"] -> _
                                frame False {
                                n3102 = local read "风机继电器"() -> (w4171:bool)
                                n3103 = Number To Hexadecimal String(2:w4175) -> (0:w4174:string)  [unwired: 1 out]
                                n3104 = local write "继电器超时处理"(TRUE ("继电器超时处理")) -> ()
                                n3105 = Not(x=w4171) -> (.not. x?=w4172:bool)
                                n3106 = Concatenate Strings("继电器操作失败,0x" ("消息"), w4174) -> (w4173:string)
                                n3107 = local write "风机继电器"(w4172) -> ()
                                }
                                frame True {
                                }
                              }
                            }
                            frame 7 {
                              n3108 = Equal To 0?(x=w4179) -> (x = 0?=w4178:bool)
                              n3109 = case shown="假" w4178 {
                                tunnel: w4179 -> [w4184 _]
                                tunnel: [w4182 "继电器操作成功!\n继电器操作成功!\n继电器操作成功!"] -> _
                                frame False {
                                n3110 = local read "加热继电器(从)"() -> (w4180:bool)
                                n3111 = Number To Hexadecimal String(2:w4184) -> (0:w4183:string)  [unwired: 1 out]
                                n3112 = Not(x=w4180) -> (.not. x?=w4181:bool)
                                n3113 = Concatenate Strings("继电器操作失败,0x" ("消息"), w4183) -> (w4182:string)
                                n3114 = local write "加热继电器(从)"(w4181) -> ()
                                }
                                frame True {
                                n3115 = local write "继电器超时处理"(TRUE ("继电器超时处理")) -> ()
                                }
                              }
                              n3116 = local write "正级继电器 7"(w4178) -> ()
                            }
                            frame 8 {
                              n3117 = Equal To 0?(x=w4189) -> (x = 0?=w4188:bool)
                              n3118 = case shown="假" w4188 {
                                tunnel: w4189 -> [w4194 _]
                                tunnel: [w4192 "继电器操作成功!\n继电器操作成功!\n继电器操作成功!"] -> _
                                frame False {
                                n3119 = local read "风机继电器(从)"() -> (w4190:bool)
                                n3120 = Number To Hexadecimal String(2:w4194) -> (0:w4193:string)  [unwired: 1 out]
                                n3121 = Not(x=w4190) -> (.not. x?=w4191:bool)
                                n3122 = Concatenate Strings("继电器操作失败,0x" ("消息"), w4193) -> (w4192:string)
                                n3123 = local write "风机继电器(从)"(w4191) -> ()
                                }
                                frame True {
                                n3124 = local write "继电器超时处理"(TRUE ("继电器超时处理")) -> ()
                                }
                              }
                              n3125 = local write "正级继电器 8"(w4188) -> ()
                            }
                            frame 85, 170 {
                              n3126 = local write "继电器超时处理"(TRUE ("继电器超时处理")) -> ()
                            }
                          }
                        }
                        frame 2 {
                          n3127 = Index Array(array=w4204) -> (element #1=w4203:u8, element #2=w4202:u8, element #3=w4201:u8)  [unwired: 3 in]
                          n3128 = Join Numbers(hi=w4202, lo=w4201) -> ((hi.lo)=w4200:u16)
                          n3129 = case shown="2" w4203 {
                            tunnel: w4204 -> [_ _ _]
                            tunnel: w4200 -> [_ w4208 w4222]
                            tunnel: w4199 -> [_ w4207 _]
                            frame 0, Default {
                              n3130 = local write "继电器超时处理"(FALSE ("继电器超时处理")) -> ()
                            }
                            frame 1 {
                              n3131 = Equal To 0?(x=w4208) -> (x = 0?=w4206:bool)
                              n3132 = case shown="假" w4206 {
                                tunnel: w4208 -> [w4214 _]
                                tunnel: [w4212 "DO控制操作成功!\nDO控制操作成功!\nDO控制操作成功!"] -> _
                                tunnel: w4207 -> [w4211 _]
                                frame False {
                                n3133 = case shown="\"主板\", 默认" w4211 {
                                frame "主板", Default {
                                n3134 = local read "DO1"() -> (w4217:bool)
                                n3135 = Not(x=w4217) -> (.not. x?=w4216:bool)
                                n3136 = local write "DO1"(w4216) -> ()
                                }
                                frame "从板" {
                                n3137 = local read "DO1 2"() -> (w4219:bool)
                                n3138 = Not(x=w4219) -> (.not. x?=w4218:bool)
                                n3139 = local write "DO1 2"(w4218) -> ()
                                }
                                }
                                n3140 = Number To Hexadecimal String(2:w4214) -> (0:w4213:string)  [unwired: 1 out]
                                n3141 = Concatenate Strings("DO控制操作失败,0x" ("消息"), w4213) -> (w4212:string)
                                }
                                frame True {
                                }
                              }
                              n3142 = case shown="\"从板\"" w4207 {
                                tunnel: w4206 -> [w4209 w4210]
                                frame "主板", Default {
                                n3143 = local write "正级继电器 9"(w4209) -> ()
                                }
                                frame "从板" {
                                n3144 = local write "正级继电器 11"(w4210) -> ()
                                }
                              }
                            }
                            frame 2 {
                              n3145 = Equal To 0?(x=w4222) -> (x = 0?=w4221:bool)
                              n3146 = case shown="假" w4221 {
                                tunnel: w4222 -> [w4227 _]
                                tunnel: [w4225 "DO控制操作成功!\nDO控制操作成功!\nDO控制操作成功!"] -> _
                                frame False {
                                n3147 = Number To Hexadecimal String(2:w4227) -> (0:w4226:string)  [unwired: 1 out]
                                n3148 = local read "DO2"() -> (w4224:bool)
                                n3149 = Not(x=w4224) -> (.not. x?=w4223:bool)
                                n3150 = Concatenate Strings("DO控制操作失败,0x" ("消息"), w4226) -> (w4225:string)
                                n3151 = local write "DO2"(w4223) -> ()
                                }
                                frame True {
                                }
                              }
                              n3152 = local write "正级继电器 10"(w4221) -> ()
                            }
                          }
                        }
                      }
                      n3153 = local write "消除"(FALSE ("消除")) -> ()
                      n3154 = global write "EV05全局变量1.vi" "流控帧 2"(FALSE ("流控帧 2")) -> ()
                      n3155 = local write "控制1"(FALSE ("控制1")) -> ()
                      "继电器超时处理" <- TRUE ("控制1")
                    }
                  }
                }
                frame "高压板校正" {
                  n3156 = local read "命令序号"() -> (w4234:u8)
                  n3157 = call "多帧接收机制(EV05).vi"("can卡类型"=w4241, "设备索引号"=w4240, "CAN端口"=w4239, "VCI_Receive"=w4238, "命令"=w4236, "板号"=w4237, "命令序号"=w4234) -> ("错误信号"=w4230:bool, "错误代码"=w4243:i32, "输出数组"=w4235:u8[], "读错误代码"=w4233:u8[], "结束信号"=w4242:bool)  [unwired: 1 in, 7 out]
                  n3158 = local read "控制1"() -> (w4231:bool)
                  n3159 = And(x=w4231, y=w4242) -> (x .and. y?=w4232:bool)
                  n3160 = case shown="真" w4232 {
                    tunnel: w4244 -> [_ w4248]
                    tunnel: w4243 -> [_ _]
                    tunnel: w4235 -> [_ w4246]
                    tunnel: w4234 -> [_ w4247]
                    tunnel: w4233 -> [_ w4249]
                    tunnel: w4230 -> [_ w4250]
                    frame False {
                    }
                    frame True {
                      n3161 = case shown="假" w4250 {
                        tunnel: w4249 -> [_ w4460]
                        tunnel: w4248 -> [_ _]
                        tunnel: w4247 -> [w4255 _]
                        tunnel: w4246 -> [w4254 _]
                        frame False {
                          n3162 = case shown="2" w4255 {
                            tunnel: w4254 -> [_ w4260 w4294 w4324 w4351 w4378 w4405 w4432]
                            frame 0, Default {
                            }
                            frame 1 {
                              n3163 = for {
                                N: 10 -> [_]
                                tunnel: w4260 -> [w4277]
                                shift-right: [w4264] -> w4258
                                shift-left: string[] [] -> [w4266]
                                i -> [w4263]
                                w4271 = 8 ("索引")
                                w4275 = 2 ("y")
                                n3164 = Multiply(x=w4263, y=w4275) -> (x*y=w4276:i32)
                                n3165 = Array Subset(array=w4277, index=w4276, length=w4275) -> (w4274:u8[])
                                n3166 = Index Array(array=w4274) -> (element #1=w4273:u8, element #2=w4272:u8)  [unwired: 2 in]
                                n3167 = call "二进制解析-8.6.vi"("索引"=w4271, "数值"=w4273) -> ("低位子数组"=w4270:i32[])  [unwired: 1 in, 2 out]
                                n3168 = call "二进制解析-8.6.vi"("索引"=w4271, "数值"=w4272) -> ("低位子数组"=w4269:i32[])  [unwired: 1 in, 2 out]
                                n3169 = Insert Into Array(array=w4270, new element=w4269) -> (w4268:i32[])  [unwired: 1 in]
                                n3170 = case shown="2" w4263 {
                                tunnel: [6 15 9 4 2 0 2] -> w4262
                                frame 0, Default {
                                }
                                frame 1 {
                                }
                                frame 2 {
                                }
                                frame 3..5 {
                                }
                                frame 8, 9 {
                                }
                                frame 7 {
                                }
                                frame 6 {
                                }
                                }
                                n3171 = Reverse 1D Array(array=w4268) -> (reversed array=w4267:i32[])
                                n3172 = for {
                                N: w4262 -> [_]
                                tunnel: w4267 -> [w4289] mode=indexing
                                tunnel: [w4285] -> w4265 mode=indexing
                                n3173 = Equal To 0?(x=w4289) -> (x = 0?=w4288:bool)
                                n3174 = Select(t="无", s=w4288, f="故障") -> (s? t:f=w4285:string)
                                }
                                n3175 = Insert Into Array(array=w4266, new element=w4265) -> (w4264:string[])  [unwired: 1 in]
                              }
                              n3176 = call "详细故障分解.vi"("名称"=string[] ["上电自检异常(CellV)", "通讯异常(CellV)", "不更新(CellV)", "未校准(CellV)", "保留", "采样线路断路(CellV)", "18b20上电自检异常(T) ", "18b20通讯异常(T)", "18b20传感器丢失(T)", "18b20传感器无号(T)", "18b20温度异常跳变(T)", "18b20信号线对电源短路(T)", "18b20信号线对地短路(T)", "18b20 CRC校验异常(T)", "NTC上电自检异常(T)", "NTC通讯异常(T)", "NTC传感器丢失(T)", "NTC温度异常跳变(T)", "NTC信号线断路(T)", "NTC信号线对电源短(T)", "NTC信号线对地短路(T)", "上电自检异常(Curr)", "参数异常(Curr)", "不更新(Curr)", "未校准(Curr)", "采样线断开(Curr)", "电流零漂异常(Curr)", "传感器反接(Curr)", "读取实时电流故障(Curr)", "平均电流故障(Curr)", "自检异常(iso)", "前端检测电阻损坏(iso)", "不更新(iso)", "未校准(iso)", "上电自检异常(Sumv_in)", "通讯异常(Sumv_in)", "不更新(Sumv_in)", "未校准(Sumv_in)", "上电自检异常(Sumv_out)", "通讯异常(Sumv_out)", "不更新(Sumv_out)", "未校准(Sumv_out)", "系统时钟自检异常(Clock)", "系统时钟未校准(Clock)", "充电均衡模块不能开启", "充电均衡模块不能关闭", "放电均衡模块不能开启", "放电均衡模块不能关闭"], "故障输入口"=w4258) -> ("输出数组"=w4256:string[][])  [unwired: 1 in, 2 out]
                              n3177 = local write "电池故障"(w4256) -> ()
                            }
                            frame 2 {
                              n3178 = for {
                                N: 5 -> [_]
                                tunnel: w4294 -> [w4311]
                                shift-right: [w4298] -> w4292
                                shift-left: string[] [] -> [w4300]
                                i -> [w4296]
                                w4305 = 8 ("索引")
                                w4309 = 2 ("y")
                                n3179 = Multiply(x=w4296, y=w4309) -> (x*y=w4310:i32)
                                n3180 = Array Subset(array=w4311, index=w4310, length=w4309) -> (w4308:u8[])
                                n3181 = Index Array(array=w4308) -> (element #1=w4307:u8, element #2=w4306:u8)  [unwired: 2 in]
                                n3182 = call "二进制解析-8.6.vi"("索引"=w4305, "数值"=w4307) -> ("低位子数组"=w4304:i32[])  [unwired: 1 in, 2 out]
                                n3183 = call "二进制解析-8.6.vi"("索引"=w4305, "数值"=w4306) -> ("低位子数组"=w4303:i32[])  [unwired: 1 in, 2 out]
                                n3184 = Insert Into Array(array=w4304, new element=w4303) -> (w4302:i32[])  [unwired: 1 in]
                                n3185 = case shown="2" w4296 {
                                tunnel: [4 6 5] -> w4297
                                frame 0, Default {
                                }
                                frame 2 {
                                }
                                frame 4 {
                                }
                                }
